vi "XY Graph Set Cursor Style 2.vi"(8 "Error In":errorcluster, 9 "Cursor Style":T1={"Cursor Point Style"=1, "Cursor Style"=8, "Line Style"=2, "Line Width"=0, "Cursor Color"=16448250} {"Cursor Color" format="%.0x"}, 10 "Cursor Idx (-1: last)":i32=-1, 11 "XYGraph in":refnum<vi>) -> (0 "Error Out":errorcluster, 3 "Vertices":cluster{"X":dbl, "Y":dbl}[](array[cluster]))   [LabVIEW 2021, in "XY Graph Add-Ons.lvlib"]
uses:
  XY Graph Add-Ons.lvlib
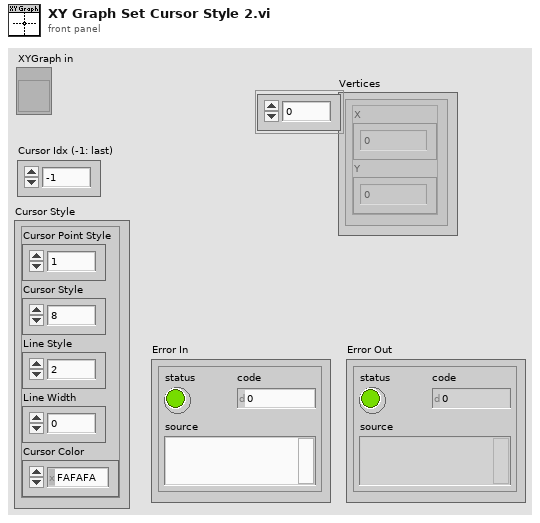
[diagram p1: front panel]
types:
  T1 = cluster{"Cursor Point Style":u8, "Cursor Style":u8, "Line Style":u8, "Line Width":u8, "Cursor Color":u32}
  T2 = typedef "LVCursorListTypeDef.ctl" = cluster{"Name":string, "Color":u32, "Style":u8, "Point Style":u8, "Name Visible":bool, "Allow Drag":bool, "Cursor Mode":u32, "Plot":i32, "Index":i32, "Position":cluster{"X":dbl, "Y":dbl}, "X Scale":u32, "Y Scale":u32, "Watch Plots":i32[], "Watch All Plots":bool, "Plot Area":i32, "Label Offset":cluster{"X":dbl, "Y":dbl}}[]
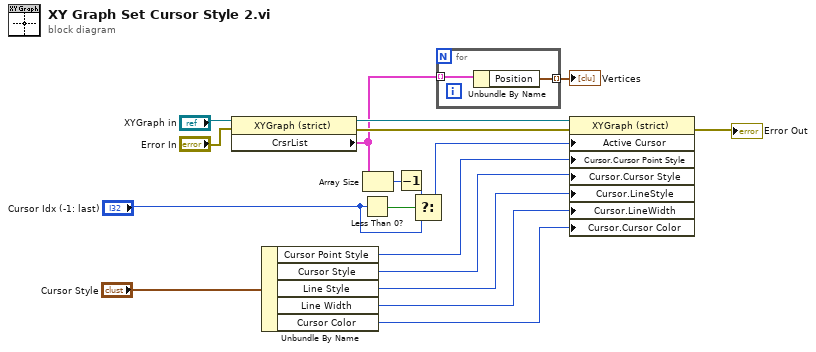
[diagram p0: block diagram]
diagram:
  n1 = property class="XYGraph (strict)"(reference="XYGraph in", error in="Error In") -> (reference out=w17:refnum<vi>, error out=w15:errorcluster, "CrsrList"=w2:T2)
  n2 = Unbundle By Name("Cursor Style") -> ("Cursor Point Style"=w9:u8, "Cursor Style"=w8:u8, "Line Style"=w7:u8, "Line Width"=w6:u8, "Cursor Color"=w5:u32)
  n3 = Less Than 0?(x="Cursor Idx (-1: last)") -> (x < 0?=w14:bool)
  n4 = Array Size(array=w2) -> (size(s)=w16:i32)
  n5 = Decrement(x=w16) -> (x-1=w13:i32)
  n6 = Select(t=w13, s=w14, f="Cursor Idx (-1: last)") -> (s? t:f=w11:i32)
  n7 = for {
    tunnel: w2 -> [w20] mode=indexing
    tunnel: [w19] -> w1 mode=indexing
    n8 = Unbundle By Name(w20) -> ("Position"=w19:cluster{"X":dbl, "Y":dbl})
  }
  "Vertices" <- w1
  n9 = property class="XYGraph (strict)"(reference=w17, error in=w15, "Active Cursor"=w11, "Cursor.Cursor Point Style"=w9, "Cursor.Cursor Style"=w8, "Cursor.LineStyle"=w7, "Cursor.LineWidth"=w6, "Cursor.Cursor Color"=w5) -> (error out=→"Error Out":errorcluster)  [unwired: 1 out]
